vi "GUI_GaugeControl.vi"() -> ()   [LabVIEW 2013]
uses:
  Shared/GUI_Template/GUI_master/tcp_new_data_event.ctl
  Shared/GUI_Template/GUI_master/tcp new data cluster.ctl
panel:
  in  "stop":bool
  in  "pressure::1":dbl caption="Pressure" min=-100.0 max=500.0
  in  "GUIdevice 1":string="P2_PDR2000"
  out "tcp data event":T1
  out "error IO 2":errorcluster
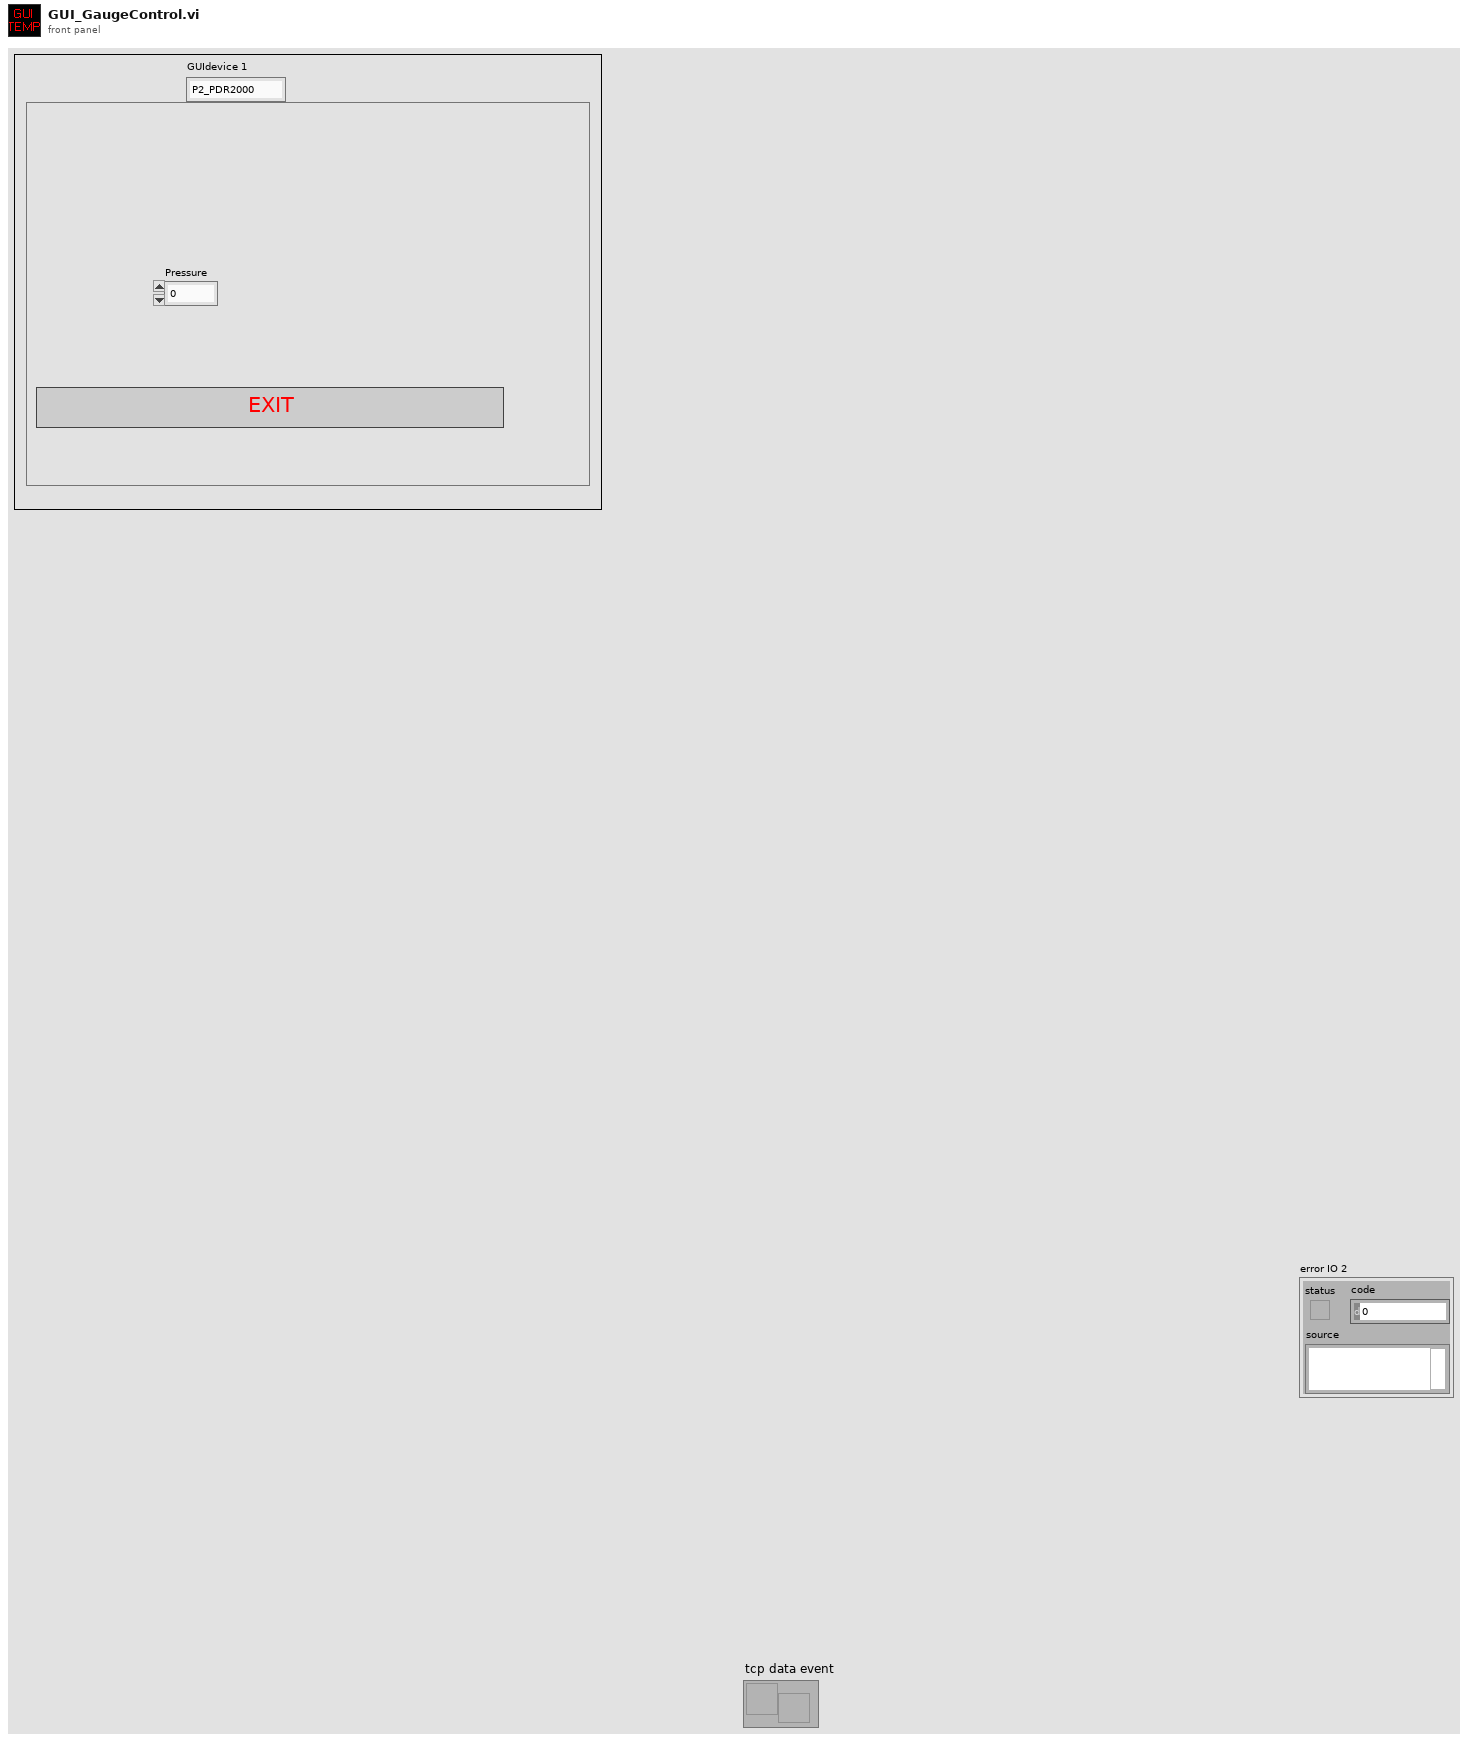
[diagram p1: front panel]
types:
  T1 = typedef "tcp_new_data_event.ctl" = refnum<user-event>
  T2 = typedef "tcp new data cluster.ctl" = cluster{"EventEnum":enum16{"new data", "connection status update"}, "Device name":string}
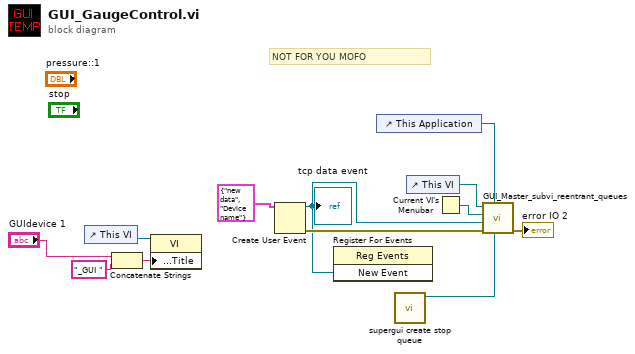
[diagram p0: block diagram]
diagram:
  # "NOT FOR YOU MOFO"
  n1 = control-ref of="This VI"() -> (w4:refnum<vi>)
  n2 = Concatenate Strings("GUIdevice 1", "_GUI ") -> (w3:string)
  n3 = property class="VI"(reference=w4, "Front Panel.Title"=w3) -> ()  [unwired: 1 in, 2 out]
  n4 = Create User Event(user event datatype=T2 {"EventEnum"=enum."new data", "Device name"="Device name"} ("New Event")) -> (user event=w7:refnum<user-event>, error out=w8:errorcluster)  [unwired: 1 in]
  "tcp data event" <- w7
  n5 = register-events(w7) -> ()  [unwired: 2 in, 2 out]
  n6 = control-ref of="This Application"() -> (w6:refnum<vi>)
  n7 = call "supergui create stop queue.vi"() -> ("STOP Queue out"=w5:refnum<queue>)  [unwired: 11 in]
  n8 = control-ref of="This VI"() -> (w11:refnum<vi>)
  n9 = Current VI's Menubar() -> (w10:refnum<k9>)
  n10 = call "GUI_Master_subvi_reentrant_queues.vi"("STOP Queue in"=w5, "This Application"=w6, "error in (no error)"=w8, "tcp data event"=w7, "Caller menu reference"=w10, "Caller VI ref"=w11) -> ("error out"=→"error IO 2":errorcluster)  [unwired: 5 in]
